vi "MathOptim-Power 2 Invert.vi"(7 "Parameters":dbl[](array[numeric]), 11 "Y":dbl format="%.2f") -> (8 "X":dbl)   [LabVIEW 2020]
doc: "This template is the starting point for creating a model function to be passed to the Nonlinear Curve Fit.vi."
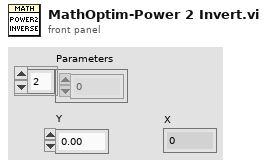
[diagram p1: front panel]
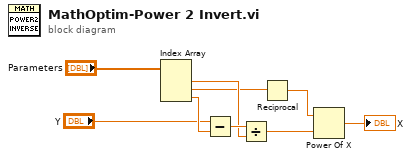
[diagram p0: block diagram]
diagram:
  n1 = Index Array(array="Parameters") -> (element #1=w5:dbl, element #2=w3:dbl, element #3=w8:dbl)  [unwired: 3 in]
  n2 = Subtract(x="Y", y=w8) -> (x-y=w6:dbl)
  n3 = Divide(x=w6, y=w5) -> (x/y=w4:dbl)
  n4 = Reciprocal(x=w3) -> (1/x=w2:dbl)
  n5 = Power Of X(1:w4, 2:w2) -> (0:→"X":dbl)
